vi "Global scelta DB rete o Locale.vi"() -> ()   [LabVIEW 2019]
panel:
  out "DB rete(F) Locale(T)":bool
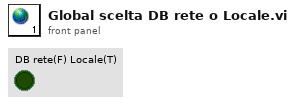
[diagram p1: front panel]
diagram:
